vi "moveabs.vi"(0 "Xpos":refnum<vi>, 1 "ZPos":refnum<vi>, 2 "YPos":refnum<vi>, 3 "ThetaPos":refnum<vi>, 5 "VISA resource name":refnum<visa-resource-name>, 7 "Theta on":bool, 9 "Y":dbl, 11 "error in (no error)":errorcluster, 12 "Z":dbl, 13 "Theta":dbl, 14 "X":dbl) -> (4 "VISA Refnum out":refnum<visa-resource-name>, 15 "error out":errorcluster)   [LabVIEW 2020]
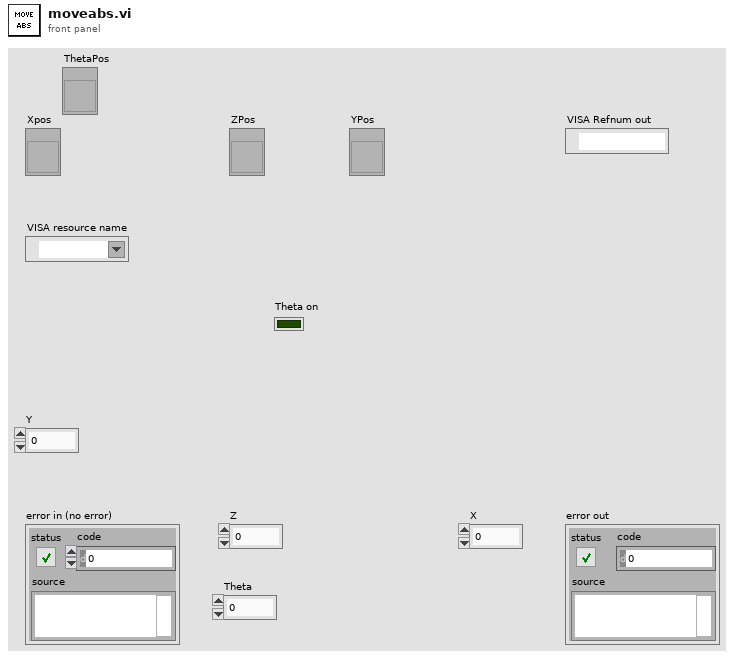
[diagram p1: front panel]
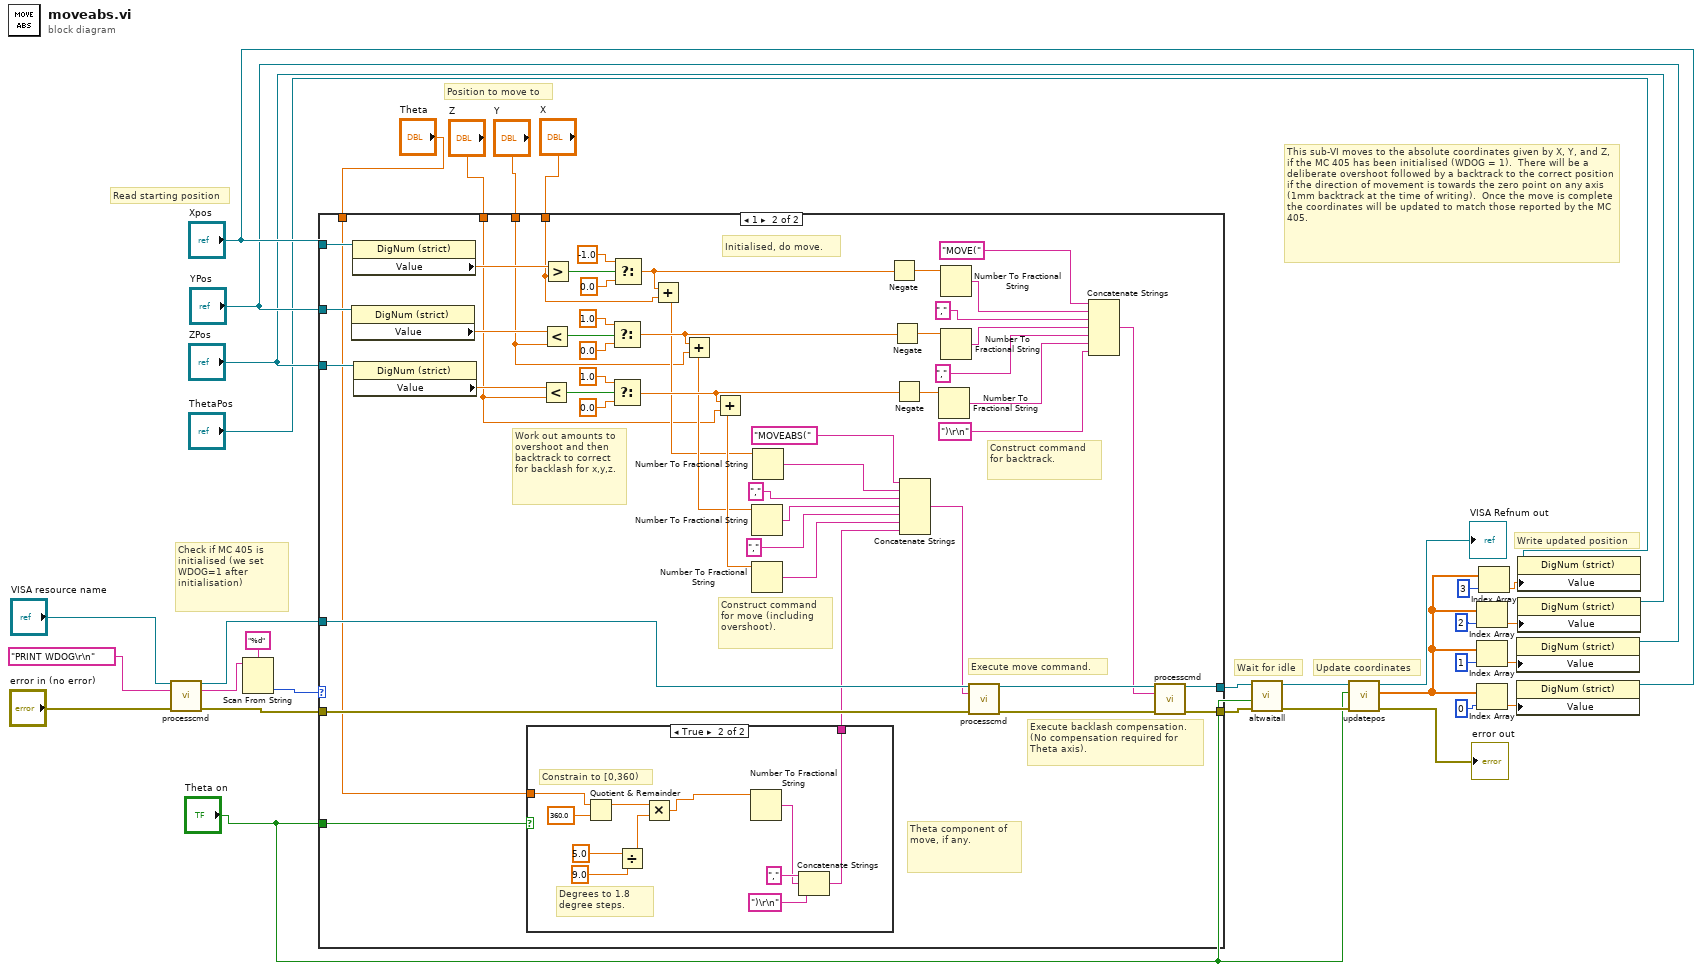
[diagram p0: block diagram]
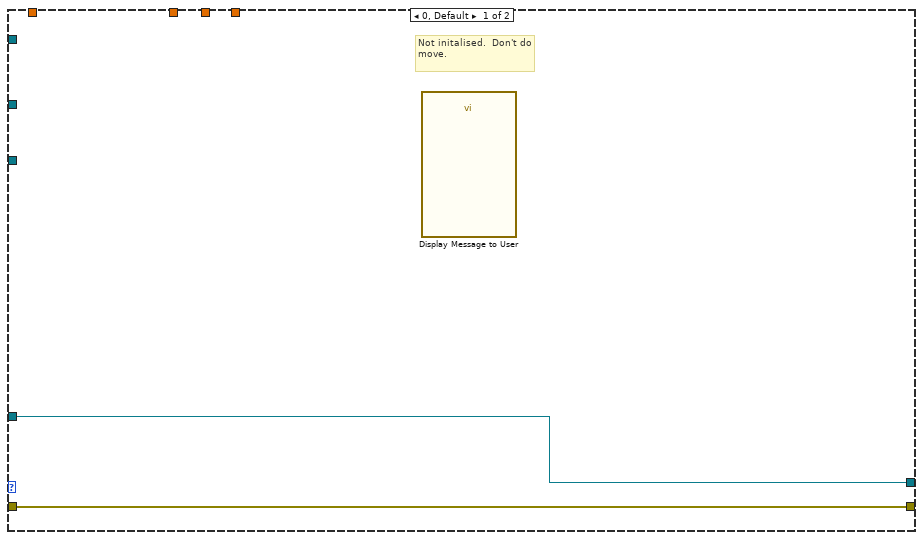
[diagram p2: hidden frame]
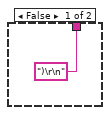
[diagram p3: hidden frame]
diagram:
  # "This sub-VI moves to the absolute coordinates given by X, Y, and Z, if the MC 405 has been initialised (WDOG = 1).  There will be a deliberate overshoot followed by a backtrack to the correct position if the direction of movement is towards the zero point on any axis (1mm backtrack at the time of writing).  Once the move is complete the coordinates will be updated to match those reported by the MC 405."
  # "Check if MC 405 is initialised (we set WDOG=1 after initialisation)"
  # "Write updated position"
  # "Read starting position"
  # "Position to move to"
  # "Update coordinates"
  # "Wait for idle"
  n1 = call "processcmd.vi"("VISA Refnum in"="VISA resource name", "write buffer"="PRINT WDOG\r\n", "error in (no error)"="error in (no error)") -> ("VISA Refnum out"=w14:refnum<visa-resource-name>, "read buffer"=w18:string, "error out"=w16:errorcluster)  [unwired: 10 in]
  n2 = Scan From String(format string="%d", input string=w18) -> (output 1=w32:i32)  [unwired: 3 in, 3 out]
  n3 = case shown="1" w32 {
    tunnel: w14 -> [w34 w85]
    tunnel: [w34 w82] -> w15
    tunnel: w16 -> [w33 w84]
    tunnel: [w33 w80] -> w17
    tunnel: "X" -> [_ w40]
    tunnel: "Y" -> [_ w39]
    tunnel: "Z" -> [_ w38]
    tunnel: "Xpos" -> [_ w43]
    tunnel: "YPos" -> [_ w42]
    tunnel: "ZPos" -> [_ w41]
    tunnel: "Theta" -> [_ w37]
    tunnel: "Theta on" -> [_ w36]
    frame 0, Default {
      # "Not initalised.  Don't do move."
      n4 = call "Display Message to User"() -> ()  [unwired: 10 in, 2 out]
    }
    frame 1 {
      # "Theta component of move, if any."
      # "Initialised, do move."
      # "Construct command for backtrack."
      # "Construct command for move (including overshoot)."
      # "Work out amounts to overshoot and then backtrack to correct for backlash for x,y,z."
      # "Execute backlash compensation.\n(No compensation required for \nTheta axis)."
      # "Execute move command."
      n5 = property class="DigNum (strict)"(reference=w42) -> ("Value"=w63:dbl)  [unwired: 1 in, 2 out]
      n6 = property class="DigNum (strict)"(reference=w43) -> ("Value"=w62:dbl)  [unwired: 1 in, 2 out]
      n7 = property class="DigNum (strict)"(reference=w41) -> ("Value"=w64:dbl)  [unwired: 1 in, 2 out]
      n8 = case shown="True" w36 {
        tunnel: w37 -> [_ w96]
        tunnel: [")\r\n" ("string") w92] -> w35
        frame False {
        }
        frame True {
          # "Degrees to 1.8 degree steps."
          # "Constrain to [0,360)"
          n9 = Quotient & Remainder(x=w96, y=360.0) -> (x-y*floor(x/y)=w91:dbl)  [unwired: 1 out]
          n10 = Divide(x=5.0, y=9.0) -> (x/y=w88:dbl)
          n11 = Multiply(x=w91, y=w88) -> (x*y=w87:dbl)
          n12 = Number To Fractional String(number=w87) -> (F-format string=w94:string)  [unwired: 3 in]
          n13 = Concatenate Strings("," ("string"), w94, ")\r\n" ("string")) -> (w92:string)
        }
      }
      n14 = Less?(x=w64, y=w38) -> (x < y?=w67:bool)
      n15 = Less?(x=w63, y=w39) -> (x < y?=w66:bool)
      n16 = Greater?(x=w62, y=w40) -> (0:w65:bool)
      n17 = Select(t=1.0, s=w66, f=0.0) -> (s? t:f=w73:dbl)
      n18 = Select(t=1.0, s=w67, f=0.0) -> (s? t:f=w74:dbl)
      n19 = Select(t=-1.0, s=w65, f=0.0) -> (s? t:f=w72:dbl)
      n20 = Add(x=w72, y=w40) -> (x+y=w68:dbl)
      n21 = Add(x=w73, y=w39) -> (x+y=w69:dbl)
      n22 = Add(x=w74, y=w38) -> (x+y=w70:dbl)
      n23 = Number To Fractional String(number=w69) -> (F-format string=w60:string)  [unwired: 3 in]
      n24 = Number To Fractional String(number=w70) -> (F-format string=w61:string)  [unwired: 3 in]
      n25 = Number To Fractional String(number=w68) -> (F-format string=w59:string)  [unwired: 3 in]
      n26 = Negate(x=w72) -> (-x=w71:dbl)
      n27 = Negate(x=w73) -> (-x=w75:dbl)
      n28 = Negate(x=w74) -> (-x=w76:dbl)
      n29 = Concatenate Strings("MOVEABS(", w59, ",", w60, ",", w61, w35) -> (w44:string)
      n30 = Number To Fractional String(number=w76) -> (F-format string=w79:string)  [unwired: 3 in]
      n31 = Number To Fractional String(number=w71) -> (F-format string=w77:string)  [unwired: 3 in]
      n32 = Number To Fractional String(number=w75) -> (F-format string=w78:string)  [unwired: 3 in]
      n33 = call "processcmd.vi"("VISA Refnum in"=w85, "write buffer"=w44, "error in (no error)"=w84) -> ("VISA Refnum out"=w83:refnum<visa-resource-name>, "error out"=w81:errorcluster)  [unwired: 10 in, 1 out]
      n34 = Concatenate Strings("MOVE(", w77, ",", w78, ",", w79, ")\r\n") -> (w45:string)
      n35 = call "processcmd.vi"("VISA Refnum in"=w83, "write buffer"=w45, "error in (no error)"=w81) -> ("VISA Refnum out"=w82:refnum<visa-resource-name>, "error out"=w80:errorcluster)  [unwired: 10 in, 1 out]
    }
  }
  n36 = call "altwaitall.vi"("error in (no error)"=w17, "Theta enabled"="Theta on", "VISA Refnum in"=w15) -> ("error out"=w19:errorcluster, "VISA Refnum out"=w20:refnum<visa-resource-name>)  [unwired: 7 in]
  n37 = call "updatepos.vi"("error in (no error)"=w19, "Theta enabled"="Theta on", "VISA Refnum in"=w20) -> ("error out"=→"error out":errorcluster, "PosArray"=w5:dbl[], "VISA Refnum out"=→"VISA Refnum out":refnum<visa-resource-name>)  [unwired: 6 in]
  n38 = Index Array(array=w5, index=2) -> (element=w21:dbl)
  n39 = Index Array(array=w5, index=1) -> (element=w22:dbl)
  n40 = Index Array(array=w5, index=0) -> (element=w23:dbl)
  n41 = Index Array(array=w5, index=3) -> (element=w2:dbl)
  n42 = property class="DigNum (strict)"(reference="YPos", "Value"=w22) -> ()  [unwired: 1 in, 2 out]
  n43 = property class="DigNum (strict)"(reference="Xpos", "Value"=w23) -> ()  [unwired: 1 in, 2 out]
  n44 = property class="DigNum (strict)"(reference="ThetaPos", "Value"=w2) -> ()  [unwired: 1 in, 2 out]
  n45 = property class="DigNum (strict)"(reference="ZPos", "Value"=w21) -> ()  [unwired: 1 in, 2 out]
